vi "get-io-names-from-tags.vi"(4 "tags":string[](array[string])) -> (1 "Array":refnum<k21>[](array[refnum]))   [LabVIEW 2015, in "dbc.lvclass"]
uses:
  dbc.lvclass
  <vilib>/xnet/xnet.llb/XNET String To IO Name (Signal).vi
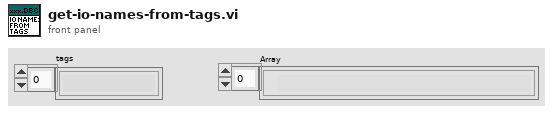
[diagram p1: front panel]
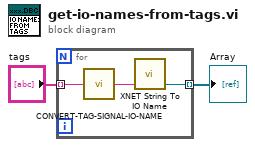
[diagram p0: block diagram]
diagram:
  n1 = for {
    tunnel: "tags" -> [w5] mode=indexing
    tunnel: [w3] -> w1 mode=indexing
    n2 = call "CONVERT-TAG-SIGNAL-IO-NAME.vi"("tag"=w5) -> ("signal"=w4:string)  [unwired: 4 in]
    n3 = call-poly <vilib>:"XNET String To IO Name.vi"("string"=w4) -> ("XNET Signal"=w3:refnum<k21>)  [unwired: 4 out]
  }
  "Array" <- w1
